vi "UI_Config.vi"() -> ()   [LabVIEW 2017]
uses:
  <vilib>/Instr/_visa.llb/VISA Configure Serial Port (Instr).vi
panel:
  in  "stop bits (10: 1 bit)":enum16{"1.0", "1.5", "2.0"}(ring)=enum."2.0" caption="停止位"
  in  "parity (0:none)":u16(ring) caption="校验" items=["None", "Odd", "Even", "Mark", "Space"]
  in  "data bits (8)":u16=8 caption="数据位" min=5 max=8 step=1
  in  "baud rate (9600)":u32=9600 caption="波特率"
  in  "Orig_Sample_Storage_Interval 10":dbl caption="转换下限阈值"
  in  "Orig_Sample_Storage_Interval 9":dbl caption="转换上限阈值"
  in  "Orig_Sample_Storage_Interval 8":dbl caption="落棒超时限值"
  in  "Orig_Sample_Storage_Interval 7":dbl caption="滤波采样窗宽"
  in  "Orig_Sample_Storage_Interval 6":dbl caption="显示更新间隔"
  in  "Orig_Sample_Storage_Interval 5":dbl caption="原始采样间隔"
  in  "Zero_Steps":bool
  in  "Orig_Sample_Storage_Interval 4":dbl caption="日志单文件大小"
  in  "Orig_Sample_Storage_Interval 3":dbl caption="采样单文件大小"
  in  "Orig_Sample_Storage_Interval 2":dbl caption="棒位单文件大小"
  in  "Orig_Sample_Storage_Interval":dbl caption="原始采样保存时间间隔"
  in  "Save_Config 3":bool
  in  "Save_Config 2":bool
  in  "Storage_Mode":enum32{"Radio Selection 1", "Radio Selection 2"}(radio)
  in  "保存内容":T1
  in  "循环次数":dbl
  in  "运行速度":dbl
  in  "Save_Config":bool
  in  "Change_Auto":bool
  in  "Single_Distance":dbl caption="单次运行距离"
  in  "Single_Step":dbl caption="单次运行步数"
  in  "Run_Mode":enum32{"Radio Selection 1", "Radio Selection 2"}(radio)
  in  "最大步位":dbl
  in  "最小步位":dbl
  in  "Init_Direction":enum32{"Radio Selection 1", "Radio Selection 2"}(radio)
  in  "初始步位":dbl
  in  "Control_Mode":enum32{"Radio Selection 1", "Radio Selection 2"}(radio)
  in  "Just_Zero":bool
  out "Run_Mode":cluster{"manual":bool, "automatic":bool}
  in  "stop":bool
  # "低温堆棒位测量试验控制系统"
  # "运行控制"
  # "存储控制"
  # "ms"
  # "MB"
  # "MB"
  # "MB"
  # "采集控制"
  # "存储方式"
  # "mm"
  # "Step"
  # "运行模式"
  # "初始运行方向"
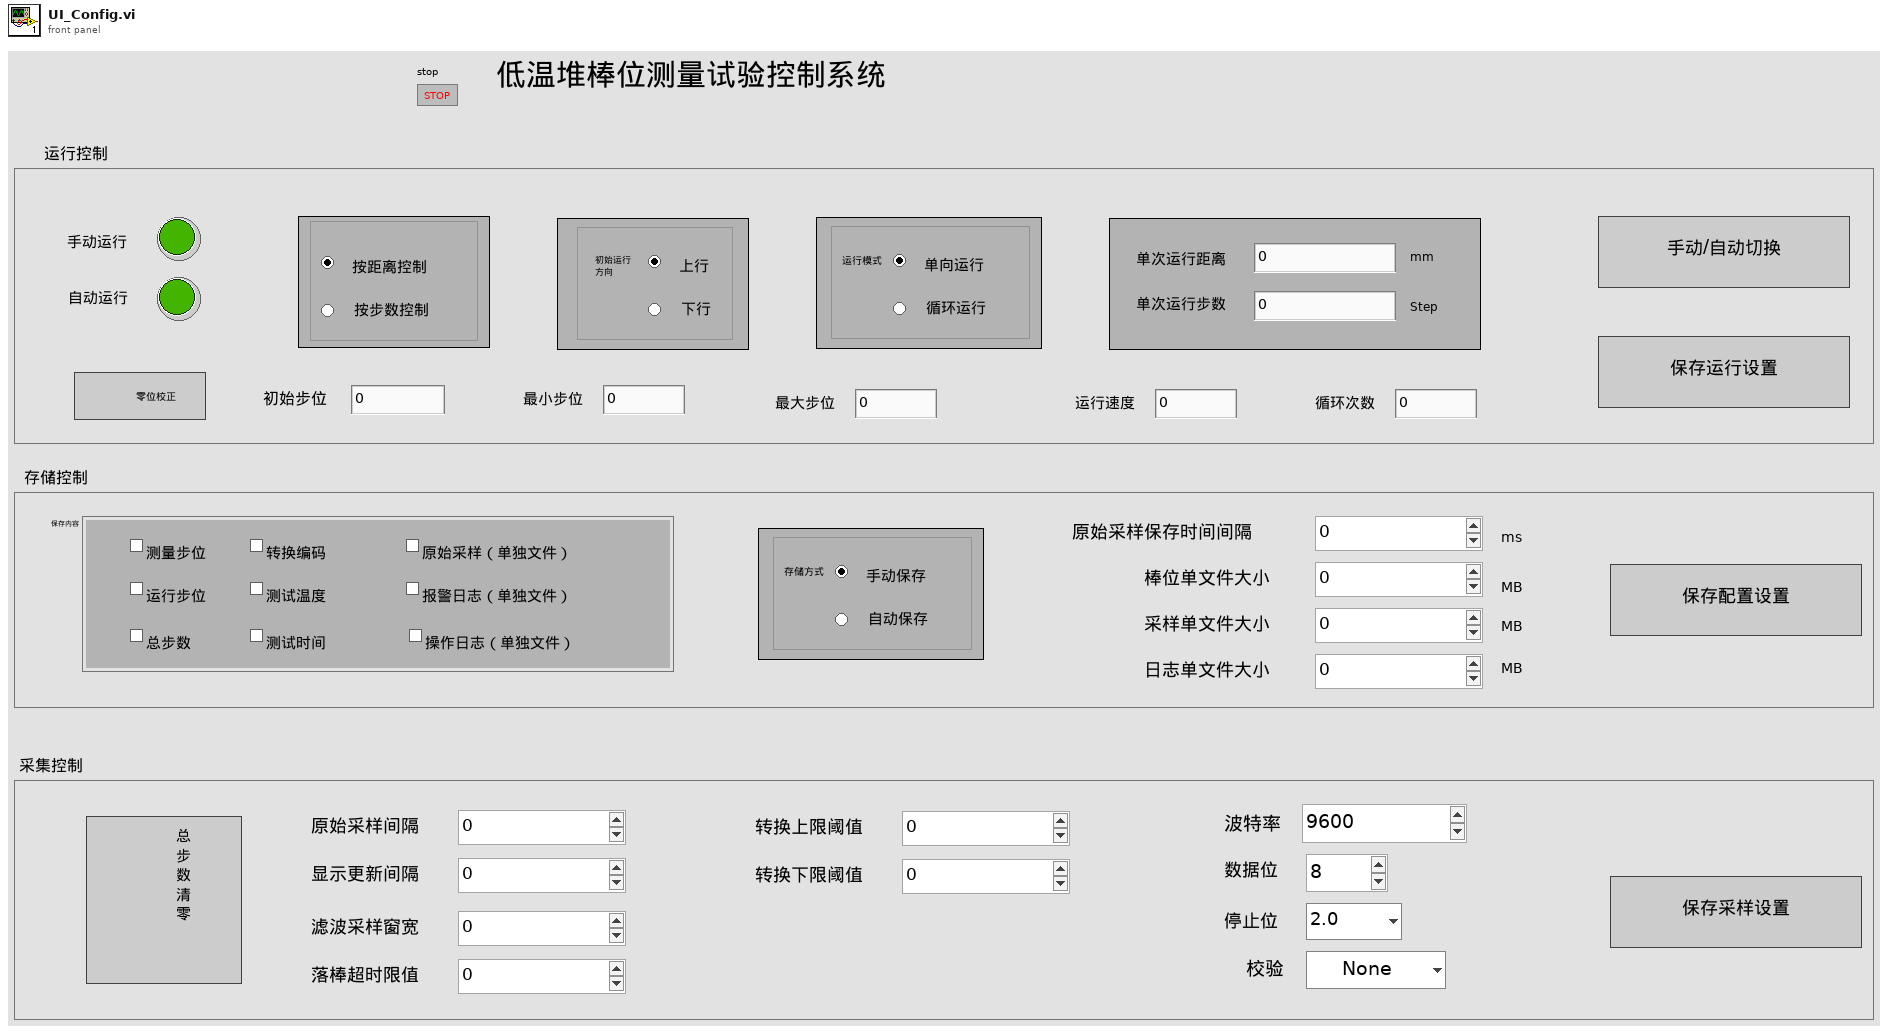
[diagram p1: front panel]
types:
  T1 = cluster{"M_Step":bool, "R_Step":bool, "Step_SUM":bool, "Conver_Code":bool, "Temperature":bool, "M_time":bool, "Orig_Sample":bool, "Alarm_log":bool, "Operate_log":bool}
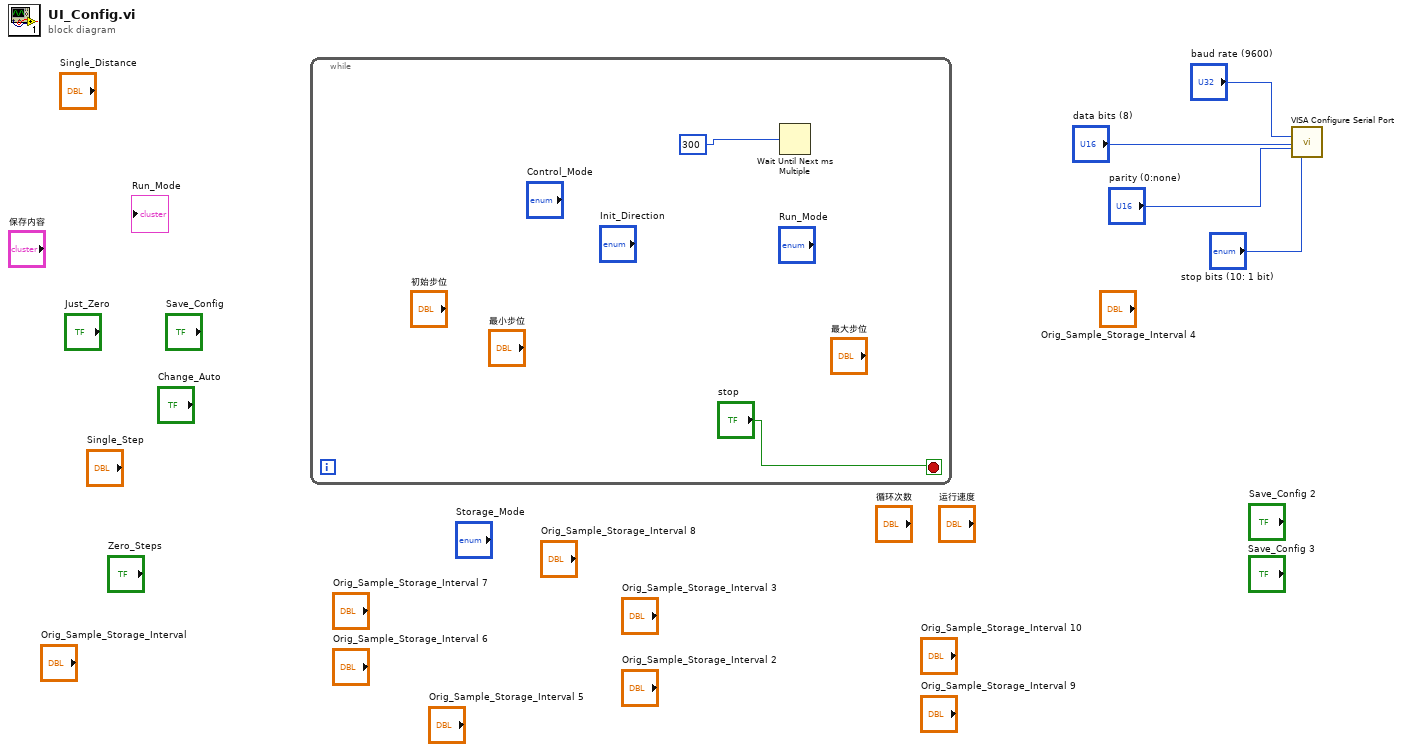
[diagram p0: block diagram]
diagram:
  n1 = while {
    stop <- "stop" stop-if-true
    n2 = Wait Until Next ms Multiple(millisecond multiple=300) -> ()  [unwired: 1 out]
  }
  n3 = call-poly "VISA Configure Serial Port"("baud rate (9600)"="baud rate (9600)", "data bits (8)"="data bits (8)", "parity (0:none)"="parity (0:none)", "stop bits (10: 1 bit)"="stop bits (10: 1 bit)") -> ()  [unwired: 10 in, 2 out]
